vi "Dashboard Main.vi"() -> ()   [LabVIEW 2015]
uses:
  AnnieFramework/DoubleSolenoidAction.ctl
  AnnieFramework/CollectorAction.ctl
  AnnieFramework/CollectorWrapAction.ctl
  AnnieFramework/CatchAction.ctl
  AnnieFramework/AutoStates.ctl
  AnnieFramework/RollerAction.ctl
  AnnieFramework/AutoMode.ctl
  AnnieFramework/PassState.ctl
  AnnieFramework/HotGoalDetectType.ctl
  AnnieFramework/LowGoalState.ctl
  <vilib>/sound2/lvsound2.llb/Sound Data Format.ctl
  TabEnum.ctl
  <vilib>/event_ctls.llb/eventvkey.ctl
  <vilib>/Rock Robotics/WPI/Dashboard/WPI_DashboardLogging Global.vi
  KariFramework/CheckImageDistance.vi
  <vilib>/Utility/config.llb/Write Key (String).vi
  <vilib>/Utility/config.llb/Write Key (I32).vi
  <vilib>/Rock Robotics/Network Tables/NT Read Boolean.vi
  <vilib>/Utility/config.llb/NI_LVConfig.lvlib
  <vilib>/sound2/lvsound2.llb/Sound Input Read (DBL).vi
  <vilib>/Analysis/NI_AALPro.lvlib
  <vilib>/sound2/lvsound2.llb/Sampling Mode.ctl
panel:
  in  "Enable Vision":bool=TRUE
  out "Image Message":string="Timeout in Camera Communications"
  in  "Rec Mode":enum32{"Stop", "Record", "Playback"}(radio)
  in  "Dashboard Tab":T1(tab)
  in  "DisableKinect":bool=TRUE
  out "Version":string
  in  "XBox":bool
  in  "DisableLCD":bool=TRUE
  out "GroundPassState":T2
  in  "DisableRollerOut":bool=TRUE
  out "FrontSonar":dbl
  out "AtPressure":bool
  out "CatchState":T3
  out "CollectorWrapState":T4
  out "CollectorState":T5
  out "CollectorMotor":dbl
  out "ClapperState":T6
  out "RollerPneuState":T6
  out "FiringCylinder2":bool
  out "FiringCylinder1":bool
  out "Kicker":bool
  out "AutoDistanceDone?":bool
  out "BackSonar":dbl
  out "BottomLS":bool
  out "TopLS":bool
  in  "MaxMotorChange":dbl=1.5
  out "Error":bool
  out "Right Motor":dbl
  out "Left Motor":dbl
  in  "Camera Settings":T7={"Frame Rate"=30, "Compression"=30, "Size"=1} {"Frame Rate" scale=1.0..30.0; "Size" items=["640x480", "320x240", "160x120"]}
  out "Mode":T8(ring)=enum.""
  out "Camera IP":string="0.0.0.11"
  in  "DB Camera Config":bool
  out "fps":dbl format="%#.1g"
  out "Mbps":dbl format="%#.1g"
  out "Mbps 2":bool
  out "Pressure":i32
  out "RollerMotorState":T9
  in  "DisableServo":bool=TRUE
  out "ElevatedPassState":T2
  out "Arcade":bool
  out "TankDriveTime":dbl
  out "SonicShifter":bool
  out "StraightDrive":bool
  out "HalfDrive":bool
  out "ReverseDrive":bool
  out "LowGoalDumpState":T10
  out "KinectTriggered?":bool
  out "ServoAngle":dbl
  out "WebcamMatched? Copy":bool
  out "PitchDetected Copy":bool
  in  "PreScumbagWait":i32
  out "CheckGoalTime":u32
  in  "StartShootTime":i32=5000
  in  "DriveBackTime":i32=1000
  in  "DriveBackSpeed":dbl=-1.0
  in  "EndInLowGear?":bool=TRUE
  out "DriveElapsedTime":u32
  in  "AccelBackward":dbl=0.1
  in  "AccelForward":dbl=0.1
  in  "StartInLowGear?":bool=TRUE
  out "ShootTime":u32
  in  "BallSettleWait":i32=130
  in  "PreCheckGoalWait":i32=260
  in  "Slowdown":dbl=36.0
  in  "Brake":dbl=12.0
  in  "DriveDistance":dbl=36.0
  in  "DriveMinTime":i32=2000
  in  "DriveTimeout":i32=4000
  out "WasHot?":bool
  out "DriveTimeOut":bool
  out "CheckGoalTimedOut?":bool
  out "ElapsedTime":u32
  out "StateTime":u32
  out "CurrentState":T11
  out "RaiseArmTimedOut":bool
  out "LowerArmTimedOut":bool
  out "IDMatched?":bool
  in  "AutoID":i32=3061
  in  "AutoMode":T12=enum."OneBallCollector"
  in  "HotGoalType":T13
  in  "ResetSound?":bool
  out "Frequency":T14(graph)={"df"=0.0, "df"=2.205, "Power Spectrum (V^2 rms)"=array[5000 elements]}
  out "RawData":waveform(dbl)[](graph)=[{"t0"=timestamp(3478468008.2170343 s since 1904-01-01), "dt"=4.5351473922902495e-05, "Y"=array[10000 elements]}, {"t0"=timestamp(3478468008.2170343 s since 1904-01-01), "dt"=4.5351473922902495e-05, "Y"=array[10000 elements]}]
  out "MaxValue":dbl=1.242701184627817e-06 format="%#.5f"
  in  "Average":dbl=1.0
  in  "Freq Bandwidth":dbl=500.0 format="%#_13g"
  in  "Start Freq":dbl=4000.0 format="%#_13g"
  in  "SoundFormat":T15={"sample rate (S/s)"=22050.0, "number of channels"=2, "bits per sample"=16}
  in  "StopSoundDetect":bool
  in  "SoundCutoff":dbl=10.0 format="%#_13g"
  out "PitchDetected":bool
  in  "% Cutoff":dbl=0.5
  out "NumHot":i32
  out "NumProcessed":i32
  in  "NumSamples":i32=5
  out "ProcessImage?":bool
  in  "Finished?":bool
  in  "Hot?":bool
  in  "Score cutoff":dbl=0.5
  in  "Color System":u16(ring)=2 items=["RGB", "HSL", "HSV", "HSI"]
  out "Distance (ft)":dbl
  in  "Color Components":T16={"Hue"={112.0, 144.0}, "Sat"={202.0, 255.0}, "Val"={237.0, 255.0}} {"Val" scale=0.0..255.0; "Sat" scale=0.0..255.0; "Hue" scale=0.0..255.0 scale format="%#_3g"}
  out "LoopTime":u32=500
  in  "Calibrate?":bool
  in  "Reset?":bool
  in  "SaveCameraImage?":bool=TRUE
  in  "TestWebcam?":bool
  in  "RunWebcam?":bool
  out "WebcamImagesProcessed":i32
  in  "ResetWebcam?":bool
  in  "WebcamImages":i32=1
  in  "SaveWebcamImage?":bool
  out "WebcamMatched?":bool
  in  "WebcamStartTime (ms)":i32=2000
  in  "StopWebcam?":bool
  out "WebcamImage":T17(plugin-control)
  in  "height":i32=480
  in  "width":i32=640
  in  "driver":i32
  in  "Test Slider":dbl(slide) scale=0.0..100.0 scale format="%#_3g"
  in  "On/Off":bool caption="Solenoid"
  in  "Test Name":u16(ring) items=["Select the test to run...", "Example Test", "-------------------------------", "List of tests is built in robot code.", "Replace with your own automated tests."]
  in  "Test Tree":string(tree)
  in  "Motor":cluster{"Value":dbl, "Enable":bool} {"Value" scale=-1.0..1.0 scale format="%#_3g"}
  out "Progress":T18 {"Test Progress" scale=0.0..100.0}
  in  "Rev/Fwd":cluster{"Forward":bool, "Reverse":bool}
  in  "Test Ring":u16(ring) items=["Auto", "Fixed indoor", "Fixed outdoor 1", "Fixed outdoor 2", "Fixed fluorescent 1", "Fixed fluorescent 2", "Hold current"]
  in  "Listbox":i32(listbox)
  out "Tree":string(tree)
  out "ClosePressure":bool
  out "CloseDist":bool
  out "FarDist":bool
  out "Timer":u32
  in  "CountdownStartTime":u32=10
  in  "AutoLength":u32=10
  in  "TeleopLength":u32=140
  out "Status":T19(ring)
  in  "Beep?":bool=TRUE
  out "SoundFilePath":path
  out "Errors":T20(array[cluster])
  in  "Reset":bool
  out "Camera Image":T17(plugin-control)
  # "DRIVE"
  # "GENERAL"
  # "OUTPUT"
  # "CONFIG"
  # "DEPRECATED"
  # "COUNTDOWN"
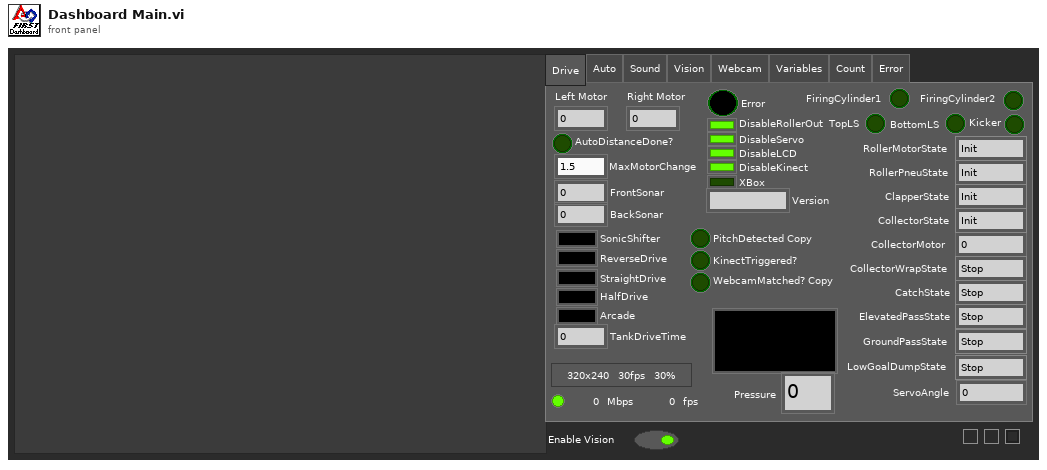
[diagram p1: front panel]
types:
  T1 = enum32{"Drive", "Auto", "Sound", "Vision", "Webcam", "Test", "Checklist", "Variables", "Count", "Error"}
  T2 = typedef "PassState.ctl" = enum16{"Stop", "Pass"}
  T3 = typedef "CatchAction.ctl" = enum16{"Stop", "PreCatch", "Catch"}
  T4 = typedef "CollectorWrapAction.ctl" = enum16{"Stop", "PreCollect", "Collect"}
  T5 = typedef "CollectorAction.ctl" = enum16{"Init", "Raise", "Lower", "Stop", "GetStatus"}
  T6 = typedef "DoubleSolenoidAction.ctl" = enum16{"Init", "Middle", "In", "Out"}
  T7 = cluster{"Frame Rate":i32, "Compression":i32, "Size":u16}
  T8 = enum8{"Tele-Op Disabled", "Tele-Op Enabled", "Auto Disabled", "Auto Enabled", "Test Disabled", "Test Enabled", ""}
  T9 = typedef "RollerAction.ctl" = enum16{"Init", "Off", "Forward", "Reverse"}
  T10 = typedef "LowGoalState.ctl" = enum16{"Stop", "Shoot"}
  T11 = typedef "AutoStates.ctl" = enum16{"Init", "LowerArmCheckGoal", "DriveBack", "Collect", "StopCollect", "LiftArm", "RaiseServo", "Drive", "ShootCollectorUp", "RaiseArm", "ShootCollectorDown", "Rotate1", "Rotate2", "Stop"}
  T12 = typedef "AutoMode.ctl" = enum16{"OneBallFront", "OneBallCollector", "TwoBallNormal", "TwoBallHot"}
  T13 = typedef "HotGoalDetectType.ctl" = enum16{"VisionTarget", "Kinect", "SoundDetect", "Webcam"}
  T14 = cluster{"df":dbl, "df":dbl, "Power Spectrum (V^2 rms)":dbl[]}
  T15 = typedef "Sound Data Format.ctl" = cluster{"sample rate (S/s)":dbl, "number of channels":i32, "bits per sample":i32}
  T16 = cluster{"Hue":cluster{dbl, dbl}, "Sat":cluster{dbl, dbl}, "Val":cluster{dbl, dbl}}
  T17 = typedef "IMAQ Image.ctl" = refnum<image>
  T18 = cluster{"Test Progress":u8, "Test Progress Text":string}
  T19 = enum8{"Disconnected", "E-Stop", "Disabled", "Enabled"}
  T20 = cluster{"status":bool, "code":i32, "location":string, "source":string}[]
  T21 = typedef "TabEnum.ctl" = enum32{"Drive", "Auto", "Sound", "Vision", "Webcam", "Variables", "Countdown", "Error"}
  T22 = typedef "Image Type" = u32
  T23 = typedef "Sampling Mode.ctl" = i32
  T24 = typedef "Sound Input Task ID.ctl" = u32
  T25 = typedef "NI_LVConfig.lvlib/Config Data RefNum.ctl" = refnum<k1>
  T26 = typedef "Sound Output Task ID.ctl" = u32
  T27 = cluster{"Digital Inputs":bool[], "Digital Outputs":bool[]}
  T28 = cluster{"Competition mode":bool, "Robot Link":bool, "Autonomous":bool, "Enabled":bool, "E-Stop":bool, "Simulated":bool, "TestMode":bool, "Docked Window":bool}
  T29 = typedef "CountdownAction.ctl" = enum16{"Start", "Reset", "Continue", "Idle"}
  T30 = cluster{"Boolean":bool, "Numeric":i32, "String":string, "String":string}[]
  T31 = cluster{cluster{dbl, dbl}, cluster{dbl, dbl}, cluster{dbl, dbl}}
  T32 = typedef "eventvkey.ctl" = enum16{"ASCII", "Enter", "Return", "Shift", "Ctrl", "Alt", "Cmd", "Opt", "Caps", "NumLock", "Clear", "Break", "Up", "Down", "Left", "Right", "Insert", "Delete", "Home", "End", "PageUp", "PageDown", "Escape", "Help", "Pause", "ScrollLock", "F1", "F2", "F3", "F4", "F5", "F6", "F7", "F8", "F9", "F10", "F11", "F12", "F13", "F14", "F15", "F16", "F17", "F18", "F19", "F20", "F21", "F22", "F23", "F24", "Play", "VolumeUp", "VolumeDown", "Mute", "Two Byte Char"}
  T33 = cluster{"Image Size":bool, "Image Type":bool, "Pixel Value":bool, "ROI Information":bool, "Zoom Factor":bool}
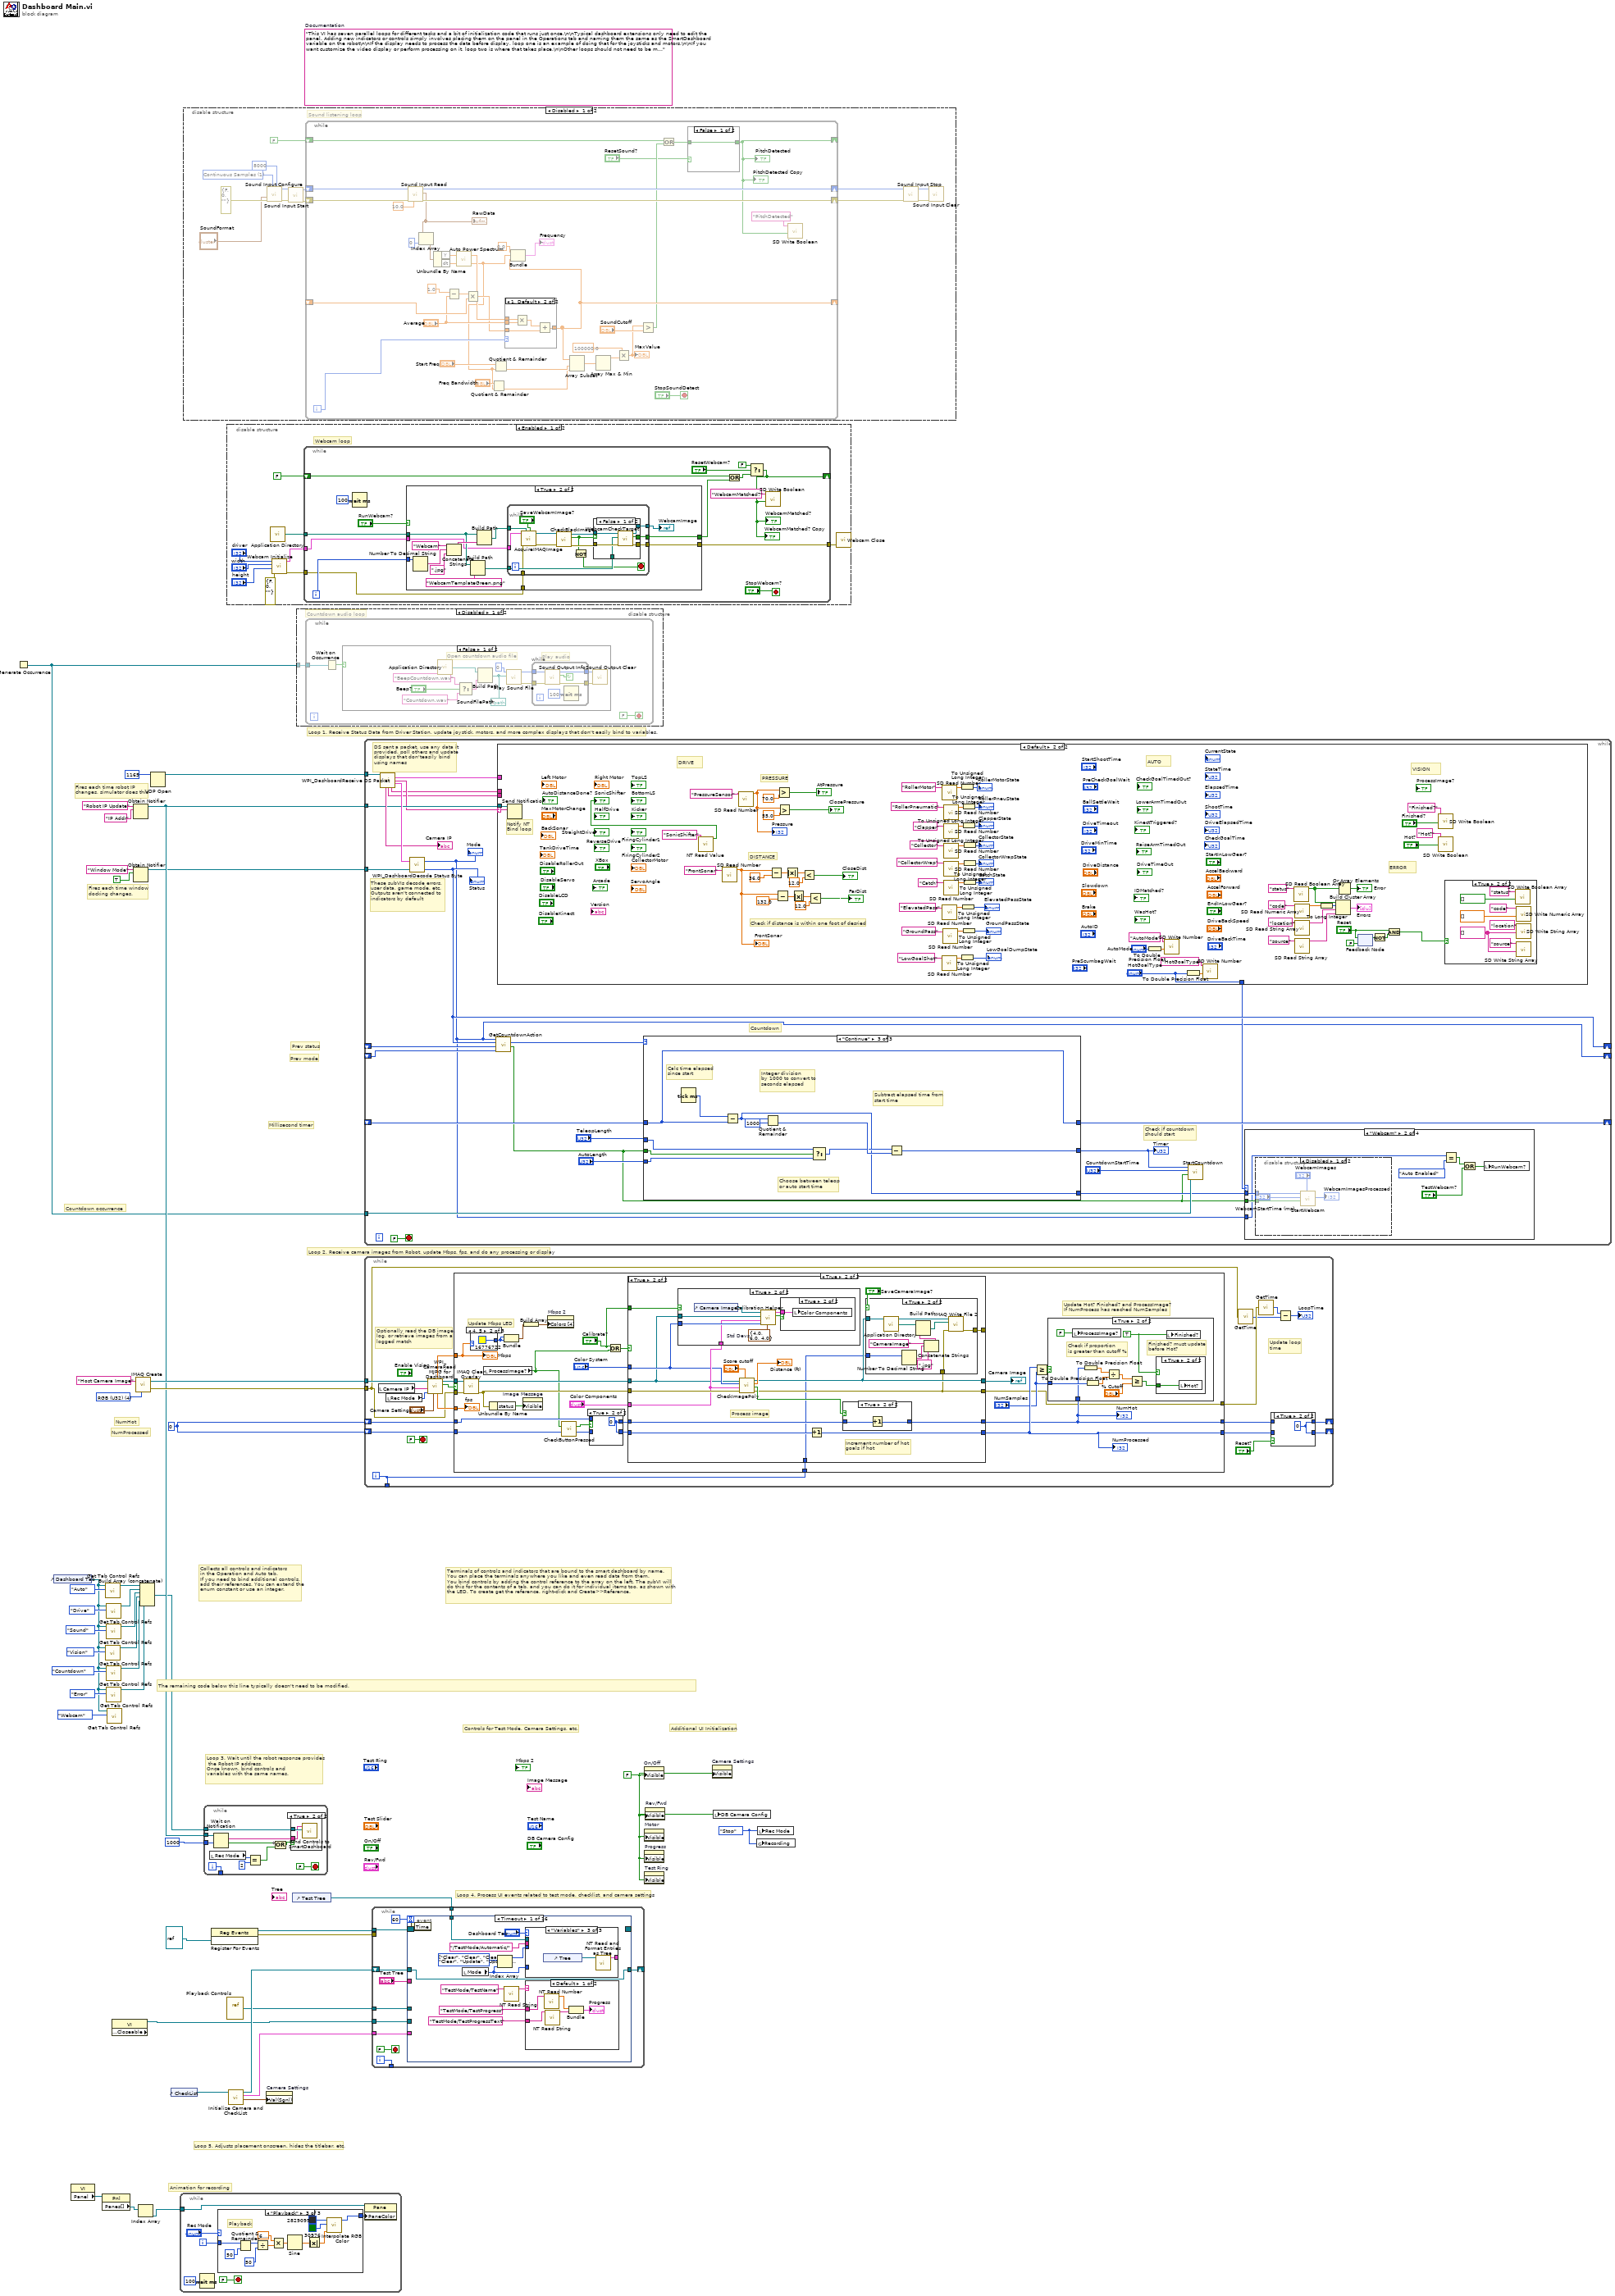
[diagram p0: block diagram]
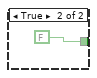
[diagram p4: hidden frame]
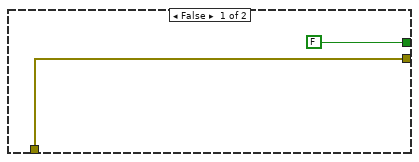
[diagram p7: hidden frame]
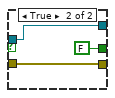
[diagram p8: hidden frame]
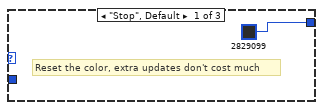
[diagram p10: hidden frame]
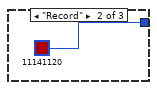
[diagram p11: hidden frame]
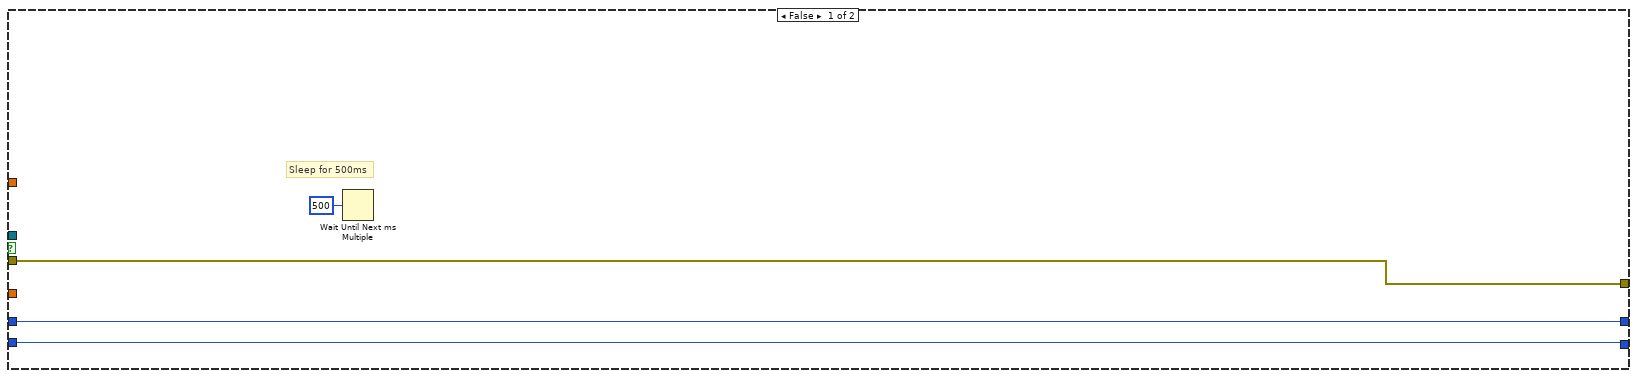
[diagram p14: hidden frame]
diagram:
  w13 = 0
  w19 = enum32{"Stop", "Record", "Playback"}."Stop" ("Rec Mode")
  w34 = FALSE ("Visible")
  (unwired) "This VI has seven parallel loops for different tasks and a bit of initialization code that runs just once.\n\nTypical dashboard extensions only need to edit the panel. Adding new indicators or controls simply involves placing them on the panel in the Operations tab and naming them the same as the SmartDashboard variable on the robot\n\nIf the display needs to process the data before display, loop one is an example of doing that for the joysticks and motors.\n\nIf you want customize the video display or perform processing on it, loop two is where that takes place.\n\nOther loops should not need to be modified. They are pretty standard, and document the task they perform."  # Documentation
  w43 = T22 4 items=["Grayscale (U8)", "Grayscale (I16)", "Grayscale (SGL)", "Complex (CSG)", "RGB (U32)", "HSL (U32)", "RGB (U64)"] ("Image Type")
  # "Prev mode"
  # "Countdown occurrence"
  # "Millisecond timer"
  # "Prev status"
  # "NumProcessed"
  # "NumHot"
  # "Controls for Test Mode, Camera Settings, etc."
  # "Additional UI Initialization"
  # "Animation for recording"
  # "Fires each time robot IP\nchanges, simulator does this"
  # "Fires each time window\ndocking changes."
  # "Collects all controls and indicators\nin the Operation and Auto tab.\nIf you need to bind additional controls,\nadd their references. You can extend the\nenum constant or use an integer."
  # "The remaining code below this line typically doesn't need to be modified."
  # "Loop 4. Process UI events related to test mode, checklist, and camera settings"
  # "Terminals of controls and indicators that are bound to the smart dashboard by name.\nYou can place the terminals anywhere you like and even read data from them.\nYou bind controls by adding the control reference to the array on the left. The subVI will\ndo this for the contents of a tab, and you can do it for individual items too, as shown with\nthe LED. To create get the reference, right-click and Create>>Reference."
  # "Loop 3. Wait until the robot response provides\n the Robot IP address.\nOnce known, bind controls and\nvariables with the same names."
  # "Loop 5. Adjusts placement onscreen, hides the titlebar, etc."
  # "Loop 1. Receive Status Data from Driver Station, update joystick, motors, and more complex displays that don't easily bind to variables."
  # "Loop 2. Receive camera images from Robot, update Mbps, fps, and do any processing or display"
  n1 = Generate Occurrence() -> (w12:refnum<k4>)
  n2 = control-ref of="Dashboard Tab"() -> (w2:refnum<vi>)
  n3 = property class="VI"() -> ("Panel"=w28:refnum<vi>)  [unwired: 2 in, 2 out]
  n4 = property class="Pnl"(reference=w28) -> ("Panes[]"=w29:refnum<vi>[])  [unwired: 1 in, 2 out]
  n5 = call <vilib>:"Get Tab Control Refs.vi"("Page Index"=TabEnum."Auto" ("Dashboard Tab"), "TabControl in"=w2) -> ("ControlsOnPage"=w17:refnum<vi>[])  [unwired: 9 in]
  n6 = call <vilib>:"Get Tab Control Refs.vi"("Page Index"=TabEnum."Vision" ("Dashboard Tab"), "TabControl in"=w2) -> ("ControlsOnPage"=w5:refnum<vi>[])  [unwired: 9 in]
  n7 = call <vilib>:"Get Tab Control Refs.vi"("Page Index"=TabEnum."Drive" ("Dashboard Tab"), "TabControl in"=w2) -> ("ControlsOnPage"=w14:refnum<vi>[])  [unwired: 9 in]
  n8 = call <vilib>:"Get Tab Control Refs.vi"("Page Index"=TabEnum."Sound" ("Dashboard Tab"), "TabControl in"=w2) -> ("ControlsOnPage"=w6:refnum<vi>[])  [unwired: 9 in]
  n9 = call <vilib>:"Get Tab Control Refs.vi"("Page Index"=TabEnum."Countdown" ("Dashboard Tab"), "TabControl in"=w2) -> ("ControlsOnPage"=w4:refnum<vi>[])  [unwired: 9 in]
  n10 = call <vilib>:"Get Tab Control Refs.vi"("Page Index"=TabEnum."Error" ("Dashboard Tab"), "TabControl in"=w2) -> ("ControlsOnPage"=w3:refnum<vi>[])  [unwired: 9 in]
  n11 = call <vilib>:"Get Tab Control Refs.vi"("Page Index"=TabEnum."Webcam" ("Dashboard Tab"), "TabControl in"=w2) -> ()  [unwired: 9 in, 1 out]
  n12 = property class="VI" props=["Front Panel.Closeable"]() -> (reference out=w18:refnum<vi>)  [unwired: 2 in, 2 out]
  n13 = Obtain Notifier(name (unnamed)="Robot IP Update", notification data type="IP Addr" ("name (unnamed)")) -> (notifier out=w37:refnum<notifier>)  [unwired: 2 in, 2 out]
  n14 = Obtain Notifier(name (unnamed)="Window Mode", notification data type=TRUE) -> (notifier out=w21:refnum<notifier>)  [unwired: 2 in, 2 out]
  n15 = call "IMAQ Create"("Image Name"="Host Camera Image", "Image Type"=w43) -> ("New Image"=w41:T17, "error out"=w40:errorcluster)  [unwired: 2 in, 1 out]
  n16 = Index Array(array=w29) -> (element=w27:refnum<vi>)  [unwired: 1 in]
  n17 = Build Array (concatenate)(w17, w14, w6, w5, w4, w3) -> (w16:refnum<vi>[])
  n18 = UDP Open(11:u16 1165 ("port")) -> (port=w44:refnum<k16>)  [unwired: 2 in, 4 out]
  n19 = control-ref of="CheckList"() -> (w20:refnum<vi>)
  n20 = while {
    tunnel: w27 -> [w47]
    i -> [w50]
    stop <- FALSE stop-if-true
    n21 = Wait (ms)(milliseconds to wait=u32 100) -> ()  [unwired: 1 out]
    n22 = case shown="\"Playback\"" "Rec Mode" {
      tunnel: w50 -> [_ _ w65]
      tunnel: [u32 2829099 ("Base Color") u32 11141120 ("Target Color") w54] -> w46
      frame "Stop", Default {
        # "Reset the color, extra updates don't cost much"
      }
      frame "Record" {
      }
      frame "Playback" {
        # "Playback"
        n23 = Quotient & Remainder(x=w65, y=u32 50 ("milliseconds to wait")) -> (x-y*floor(x/y)=w61:u32)  [unwired: 1 out]
        n24 = Divide(x=w61, y=u32 50 ("milliseconds to wait")) -> (x/y=w58:dbl)
        n25 = Multiply(x=6.283185307179586, y=w58) -> (x*y=w63:dbl)
        n26 = Sine(x=w63) -> (sin(x)=w62:dbl)
        n27 = Absolute Value(x=w62) -> (abs(x)=w55:dbl)
        n28 = call "Interpolate RGB Color.vi"("Proportion"=w55, "Target Color"=u32 30976, "Base Color"=u32 2829099) -> ("Result Color"=w54:u32)  [unwired: 8 in]
      }
    }
    n29 = property class="Pane"(reference=w47, "PaneColor"=w46) -> ()  [unwired: 1 in, 2 out]
  }
  n30 = disable-structure shown="Disabled" {
    frame Disabled {
      w77 = T23 1 items=["Finite Samples", "Continuous Samples"] ("sample mode")
      # "Sound listening loop"
      n31 = call <vilib>:"Sound Input Configure.vi"("number of samples/ch"=8000, "sample mode"=w77, "error in (no error)"=errorcluster {"status"=FALSE, "code"=0, "source"=""}, "sound format"="SoundFormat") -> ("error out"=w74:errorcluster, "task ID"=w75:T24)  [unwired: 6 in]
      n32 = call <vilib>:"Sound Input Start.vi"("error in (no error)"=w74, "task ID"=w75) -> ("error out"=w73:errorcluster, "task ID out"=w72:T24)  [unwired: 8 in]
      n33 = while {
        shift-right: [w111] -> w71
        shift-left: w73 -> [w113]
        shift-right: [w112] -> w70
        shift-left: w72 -> [w114]
        shift-right: [w108] -> _
        shift-left: _ -> [w110]
        shift-right: [w79] -> _
        shift-left: FALSE -> [w84]
        i -> [w109]
        stop <- "StopSoundDetect" stop-if-true
        n34 = call-poly <vilib>:"Sound Input Read.vi"("timeout (sec)"=10.0, "error in (no error)"=w113, "task ID"=w114) -> ("error out"=w111:errorcluster, "data"=w106:waveform(dbl)[], "task ID out"=w112:T24)  [unwired: 6 in]
        "RawData" <- w106
        n35 = Index Array(array=w106, index=0) -> (element=w102:waveform(dbl))
        n36 = Unbundle By Name(w102) -> ("Y"=w103:dbl[], "dt"=w100:dbl)
        n37 = Subtract(x=1.0, y="Average") -> (x-y=w96:dbl)
        n38 = call <vilib>:"Auto Power Spectrum.vi"("dt"=w100, "Signal (V)"=w103) -> ("df"=w92:dbl, "Power Spectrum (V^2 rms)"=w99:dbl[])
        n39 = Multiply(x=w96, y=w110) -> (x*y=w95:dbl[])
        n40 = Quotient & Remainder(x="Freq Bandwidth", y=w92) -> (floor(x/y)=w90:dbl)  [unwired: 1 out]
        n41 = Quotient & Remainder(x="Start Freq", y=w92) -> (floor(x/y)=w91:dbl)  [unwired: 1 out]
        n42 = case shown="1, Default" w109 {
          tunnel: w99 -> [w118 w123]
          tunnel: "Average" -> [_ w122]
          tunnel: w95 -> [_ w120]
          tunnel: [w118 w119] -> w108
          frame 0 {
          }
          frame 1, Default {
            n43 = Multiply(x=w123, y=w122) -> (x*y=w121:dbl[])
            n44 = Add(x=w121, y=w120) -> (x+y=w119:dbl[])
          }
        }
        n45 = Bundle("df"=0.0, "df"=w92, "Power Spectrum (V^2 rms)"=w108) -> (→"Frequency":T14)  [unwired: 1 in]
        n46 = Array Subset(array=w108, index=w91, length=w90) -> (w89:dbl[])
        n47 = Array Max & Min(array=w89) -> (max value=w88:dbl)  [unwired: 3 out]
        n48 = Multiply(x=100000.0, y=w88) -> (x*y=w85:dbl)
        "MaxValue" <- w85
        n49 = Greater?(x=w85, y="SoundCutoff") -> (0:w83:bool)
        n50 = Or(x=w84, y=w83) -> (x .or. y?=w82:bool)
        n51 = case shown="False" "ResetSound?" {
          tunnel: w82 -> [w116 _]
          tunnel: [w116 FALSE] -> w79
          frame False {
          }
          frame True {
          }
        }
        "PitchDetected" <- w79
        "PitchDetected Copy" <- w79
        n52 = call <vilib>:"SD Write Boolean.vi"("Boolean"=w79, "Name"="PitchDetected") -> ()  [unwired: 8 in, 2 out]
      }
      n53 = call <vilib>:"Sound Input Stop.vi"("error in (no error)"=w71, "task ID"=w70) -> ("error out"=w69:errorcluster, "task ID out"=w68:T24)  [unwired: 8 in]
      n54 = call <vilib>:"Sound Input Clear.vi"("error in (no error)"=w69, "task ID"=w68) -> ()  [unwired: 9 in, 1 out]
    }
    frame Enabled {
    }
  }
  n55 = while {
    tunnel: w16 -> [w134]
    tunnel: w37 -> [w132]
    tunnel: [w130] -> _
    tunnel: u32 1000 ("milliseconds to wait") -> [w129]
    i -> [w130]
    stop <- FALSE stop-if-true
    n56 = local read "Rec Mode"() -> (w125:enum32{"Stop", "Record", "Playback"})
    n57 = Wait on Notification(notifier=w132, timeout in ms (-1)=w129) -> (notification=w131:string, timed out?=w127:bool)  [unwired: 2 in, 2 out]
    n58 = Equal?(x=w125, y=u16 2 ("Rec Mode")) -> (x = y?=w126:bool)
    n59 = Compound Arithmetic op=OR(invert w127, w126) -> (w128:bool)
    n60 = case shown="True" w128 {
      tunnel: w134 -> [_ w136]
      tunnel: w131 -> [_ w135]
      frame False {
      }
      frame True {
        n61 = call <vilib>:"Bind Controls to SmartDashboard.vi"("Bound Control Refs"=w136, "Server IP Address"=w135) -> ()  [unwired: 10 in]
      }
    }
  }
  n62 = register-events(refnum<vi> refnum) -> (reference out=w25:refnum<event-registration>, error out=w24:errorcluster)  [unwired: 2 in]
  n63 = disable-structure shown="Enabled" {
    frame Enabled {
      # "Webcam loop"
      n64 = call <vilib>:"Application Directory.vi"() -> ("Application Directory"=w137:path)
      n65 = call "Webcam Initialize.vi"("error in"=errorcluster {"status"=FALSE, "code"=0, "source"=""}, "height (240)"="height", "width (320)"="width", "driver (0)"="driver") -> ("error out"=w140:errorcluster, "webcam image out"=w141:cluster{"image":u8[], "width":i32, "height":i32})  [unwired: 4 in, 1 out]
      n66 = while {
        tunnel: w137 -> [w160]
        tunnel: w141 -> [w158]
        tunnel: w140 -> [w157]
        tunnel: [w156] -> w139
        shift-right: [w146] -> _
        shift-left: FALSE -> [w152]
        i -> [w159]
        stop <- "StopWebcam?" stop-if-true
        n67 = Wait (ms)(milliseconds to wait=u32 100) -> ()  [unwired: 1 out]
        n68 = case shown="True" "RunWebcam?" {
          tunnel: [w161 w176] -> w156
          tunnel: [FALSE ("MatchFound?") w175] -> w151
          tunnel: w159 -> [_ w173]
          tunnel: w160 -> [_ w168]
          tunnel: w158 -> [_ w165]
          tunnel: w157 -> [w161 w164]
          frame False {
          }
          frame True {
            n69 = Number To Decimal String(number=w173) -> (decimal integer string=w172:string)  [unwired: 1 in]
            n70 = Concatenate Strings("Webcam", w172, ".jpg" ("string")) -> (w171:string)
            n71 = Build Path(base path=w168, name or relative path="WebcamTemplateGreen.png") -> (appended path=w167:path)
            n72 = Build Path(base path=w168, name or relative path=w171) -> (appended path=w170:path)
            n73 = while {
              tunnel: [w190] -> w176
              tunnel: [w189] -> w175
              tunnel: w170 -> [w188]
              tunnel: w167 -> [w186]
              tunnel: w165 -> [w179]
              tunnel: w164 -> [w178]
              tunnel: [w177] -> w163
              stop <- w180 stop-if-true
              n74 = call "AcquireIMAQImage.vi"("ImagePath"=w188, "SaveToDisk?"="SaveWebcamImage?", "error in"=w178, "webcam image in"=w179) -> ("error out"=w185:errorcluster, "ImageOut"=w183:T17)  [unwired: 6 in]
              n75 = call "CheckBlackImage.vi"("error in"=w185, "Image In"=w183) -> ("error out"=w184:errorcluster, "Black?"=w181:bool, "Image Out"=w182:T17)  [unwired: 7 in]
              n76 = Not(x=w181) -> (.not. x?=w180:bool)
              n77 = case shown="False" w181 {
                tunnel: w182 -> [w196 w197]
                tunnel: w184 -> [w195 w199]
                tunnel: [w194 w199] -> w190
                tunnel: [w193 FALSE ("MatchFound?")] -> w189
                tunnel: w186 -> [w192 _]
                tunnel: [w191 w197] -> w177
                frame False {
                  n78 = call "WebcamCheckTarget.vi"("error in"=w195, "TemplatePath"=w192, "ImageIn"=w196) -> ("error out"=w194:errorcluster, "MatchFound?"=w193:bool, "Image Out"=w191:T17)  [unwired: 6 in]
                }
                frame True {
                }
              }
            }
            "WebcamImage" <- w163
          }
        }
        n79 = Or(x=w152, y=w151) -> (x .or. y?=w149:bool)
        n80 = Select(t=FALSE, s="ResetWebcam?", f=w149) -> (s? t:f=w146:bool)
        "WebcamMatched?" <- w146
        "WebcamMatched? Copy" <- w146
        n81 = call <vilib>:"SD Write Boolean.vi"("Boolean"=w146, "Name"="WebcamMatched?") -> ()  [unwired: 8 in, 2 out]
      }
      n82 = call "Webcam Close.vi"("error in"=w139) -> ()  [unwired: 9 in, 1 out]
    }
    frame Disabled {
    }
  }
  n83 = vi-ref "Playback Controls.vi"() -> (w26:refnum<vi>)
  n84 = call "Initialize Camera and CheckList.vi"("ListBox in"=w20) -> ("Cluster"=w32:cluster{"value":i32, "value":i32, "index":i32}, "Array"=w33:cluster{string[]}[], "File Refnum"=w31:T25)  [unwired: 8 in]
  n85 = property on="Camera Settings" class="Clust (strict)"("Val(Sgnl)"=w32) -> ()  [unwired: 2 in, 2 out]
  n86 = control-ref of="Test Tree"() -> (w30:refnum<vi>)
  n87 = disable-structure shown="Disabled" {
    disable-tunnel: w12 -> [w200 _]
    frame Disabled {
      # "Countdown audio loop"
      n88 = while {
        tunnel: w200 -> [w201]
        stop <- FALSE stop-if-true
        n89 = Wait on Occurrence(2:w201) -> (0:w203:bool)  [unwired: 2 in]
        n90 = case shown="False" w203 {
          frame False {
            # "Play audio"
            # "Open countdown audio file"
            n91 = call <vilib>:"Application Directory.vi"() -> ("Application Directory"=w204:path)
            n92 = Select(t="BeepCountdown.wav" ("name or relative path"), s="Beep?", f="Countdown.wav" ("name or relative path")) -> (s? t:f=w206:string)
            n93 = Build Path(base path=w204, name or relative path=w206) -> (appended path=w205:path)
            "SoundFilePath" <- w205
            n94 = call <vilib>:"Play Sound File.vi"("path"=w205, "device ID"=u32 0) -> ("error out"=w213:errorcluster, "task ID"=w212:T26)  [unwired: 8 in]
            n95 = while {
              tunnel: w213 -> [w215]
              tunnel: w212 -> [w219]
              tunnel: [w218] -> w211
              tunnel: [w216] -> w210
              stop <- w217 continue-if-true
              n96 = call <vilib>:"Sound Output Info.vi"("error in (no error)"=w215, "task ID"=w219) -> ("error out"=w216:errorcluster, "is playing?"=w217:bool, "task ID out"=w218:T26)  [unwired: 6 in, 1 out]
              n97 = Wait (ms)(milliseconds to wait=u32 100) -> ()  [unwired: 1 out]
            }
            n98 = call <vilib>:"Sound Output Clear.vi"("error in (no error)"=w210, "task ID"=w211) -> ()  [unwired: 9 in, 1 out]
          }
          frame True {
          }
        }
      }
    }
    frame Enabled {
    }
  }
  n99 = while {
    tunnel: w44 -> [w243]
    tunnel: w37 -> [w240]
    tunnel: w21 -> [w242]
    shift-right: [w235] -> _
    shift-left: _ -> [w234]
    shift-right: [w232] -> _
    shift-left: _ -> [w231]
    tunnel: w12 -> [w226]
    shift-right: [w221] -> _
    shift-left: _ -> [w223]
    stop <- FALSE stop-if-true
    # "Check if countdown\nshould start"
    # "Countdown"
    # "DS sent a packet. use any data it\nprovided, poll others and update\ndisplays that don'teasily bind\nusing names"
    # "These subVIs decode errors, user data, game mode, etc.\nOutputs aren't connected to indicators by default"
    n100 = call <vilib>:"WPI_DashboardReceive DS Packet.vi"("Recv Socket"=w243) -> ("Driver Station"=w236:T27, "Robot IP Address"=w239:string, "Status"=w244:T28, "Camera IP Address"=→"Camera IP":string, "Low Priority User Data"=w238:string, "High Priority User Data"=w237:string)  [unwired: 2 in, 7 out]
    n101 = call <vilib>:"WPI_DashboardDecode Status Byte.vi"("Window Mode Notifier"=w242, "Status"=w244) -> ("Status"=w235:T19, "Mode"=w221:T8)
    "Mode" <- w221
    "Status" <- w235
    n102 = call "GetCountdownAction.vi"("PrevMode"=w223, "PrevStatus"=w234, "CurrentStatus"=w235, "CurrentMode"=w221) -> ("Teleop?"=w224:bool, "Action"=w233:T29)  [unwired: 6 in]
    n103 = case shown="Default" w239 {
      selector: w239 -> [_ w350]
      tunnel: w240 -> [_ w351]
      tunnel: w238 -> [_ _]
      tunnel: w237 -> [_ _]
      tunnel: w236 -> [_ _]
      tunnel: [_ "HotGoalType"] -> w222
      frame "0.0.0.0" {
        # "DS not sending packets, or no robot exists yet.\nDon't poll the variables"
      }
      frame Default {
        # "Check if distance is within one foot of desried"
        # "ERROR"
        # "DISTANCE"
        # "PRESSURE"
        # "VISION"
        # "AUTO"
        # "DRIVE"
        # "Notify NT\nBind loop"
        n104 = Send Notification(notification=w350, notifier=w351) -> ()  [unwired: 1 in, 2 out]
        n105 = call-poly <vilib>:"NT Read Value.vi"("Name"="SonicShifter") -> ("Boolean"=→"SonicShifter":bool)  [unwired: 9 in, 1 out]
        n106 = call <vilib>:"SD Read Number.vi"("Name"="FrontSonar") -> ("Numeric"=w301:dbl)  [unwired: 8 in, 2 out]
        "FrontSonar" <- w301
        n107 = call <vilib>:"SD Read Number.vi"("Name"="PressureSensor") -> ("Numeric"=w300:dbl)  [unwired: 8 in, 2 out]
        "Pressure" <- w300
        n108 = Subtract(x=w301, y=36.0) -> (x-y=w308:dbl)
        n109 = Subtract(x=w301, y=132.0) -> (x-y=w303:dbl)
        n110 = Greater?(x=w300, y=70.0) -> (0:→"AtPressure":bool)
        n111 = Greater?(x=w300, y=55.0) -> (0:→"ClosePressure":bool)
        n112 = Absolute Value(x=w308) -> (abs(x)=w307:dbl)
        n113 = Absolute Value(x=w303) -> (abs(x)=w304:dbl)
        n114 = Less?(x=w307, y=12.0) -> (x < y?=→"CloseDist":bool)
        n115 = Less?(x=w304, y=12.0) -> (x < y?=→"FarDist":bool)
        n116 = call <vilib>:"SD Read Number.vi"("Name"="LowGoalShot") -> ("Numeric"=w284:dbl)  [unwired: 8 in, 2 out]
        n117 = call <vilib>:"SD Read Number.vi"("Name"="RollerMotor") -> ("Numeric"=w298:dbl)  [unwired: 8 in, 2 out]
        n118 = call <vilib>:"SD Read Number.vi"("Name"="ElevatedPass") -> ("Numeric"=w292:dbl)  [unwired: 8 in, 2 out]
        n119 = call <vilib>:"SD Read Number.vi"("Name"="GroundPass") -> ("Numeric"=w291:dbl)  [unwired: 8 in, 2 out]
        n120 = call <vilib>:"SD Read Number.vi"("Name"="RollerPneumatic") -> ("Numeric"=w328:dbl)  [unwired: 8 in, 2 out]
        n121 = call <vilib>:"SD Read Number.vi"("Name"="Clapper") -> ("Numeric"=w326:dbl)  [unwired: 8 in, 2 out]
        n122 = call <vilib>:"SD Read Number.vi"("Name"="Collector") -> ("Numeric"=w323:dbl)  [unwired: 8 in, 2 out]
        n123 = call <vilib>:"SD Read Number.vi"("Name"="CollectorWrap") -> ("Numeric"=w320:dbl)  [unwired: 8 in, 2 out]
        n124 = call <vilib>:"SD Read Number.vi"("Name"="Catch") -> ("Numeric"=w317:dbl)  [unwired: 8 in, 2 out]
        n125 = To Unsigned Long Integer(number=w298) -> (unsigned 32bit integer=→"RollerMotorState":u32)
        n126 = To Unsigned Long Integer(number=w284) -> (unsigned 32bit integer=→"LowGoalDumpState":u32)
        n127 = To Unsigned Long Integer(number=w292) -> (unsigned 32bit integer=→"ElevatedPassState":u32)
        n128 = To Unsigned Long Integer(number=w328) -> (unsigned 32bit integer=→"RollerPneuState":u32)
        n129 = To Unsigned Long Integer(number=w326) -> (unsigned 32bit integer=→"ClapperState":u32)
        n130 = To Unsigned Long Integer(number=w291) -> (unsigned 32bit integer=→"GroundPassState":u32)
        n131 = To Unsigned Long Integer(number=w323) -> (unsigned 32bit integer=→"CollectorState":u32)
        n132 = To Unsigned Long Integer(number=w320) -> (unsigned 32bit integer=→"CollectorWrapState":u32)
        n133 = To Unsigned Long Integer(number=w317) -> (unsigned 32bit integer=→"CatchState":u32)
        n134 = To Double Precision Float(number="AutoMode") -> (double precision float=w294:dbl)
        n135 = call <vilib>:"SD Write Number.vi"("Numeric"=w294, "Name"="AutoMode") -> ()  [unwired: 8 in, 2 out]
        n136 = To Double Precision Float(number="HotGoalType") -> (double precision float=w287:dbl)
        n137 = call <vilib>:"SD Write Number.vi"("Numeric"=w287, "Name"="HotGoalType") -> ()  [unwired: 8 in, 2 out]
        n138 = call <vilib>:"SD Read Boolean Array.vi"("Name"="status") -> ("Boolean Array"=w339:bool[])  [unwired: 8 in, 2 out]
        n139 = call <vilib>:"SD Read Numeric Array.vi"("Name"="code") -> ("Numeric Array"=w338:dbl[])  [unwired: 8 in, 2 out]
        n140 = call <vilib>:"SD Read String Array.vi"("Name"="location") -> ("String Array"=w337:string[])  [unwired: 9 in, 1 out]
        n141 = call <vilib>:"SD Read String Array.vi"("Name"="source") -> ("String Array"=w336:string[])  [unwired: 9 in, 1 out]
        n142 = To Long Integer(number=w338) -> (32bit integer=w344:i32[])
        n143 = Build Cluster Array(w339, w344, w337, w336) -> (→"Errors":T30)
        n144 = Or Array Elements(Boolean array=w339) -> (logical OR=→"Error":bool)
        n145 = feedback #1(FALSE ("Reset")) -> (w347:bool)
        n146 = feedback-in #1("Reset") -> ()
        n147 = Not(x=w347) -> (.not. x?=w346:bool)
        n148 = And(x="Reset", y=w346) -> (x .and. y?=w345:bool)
        n149 = call <vilib>:"SD Write Boolean.vi"("Boolean"="Finished?", "Name"="Finished?") -> ()  [unwired: 8 in, 2 out]
        n150 = call <vilib>:"SD Write Boolean.vi"("Boolean"="Hot?", "Name"="Hot?") -> ()  [unwired: 8 in, 2 out]
        n151 = case shown="True" w345 {
          frame False {
          }
          frame True {
            w352 = string[] [] ("String Array")
            n152 = call <vilib>:"SD Write Boolean Array.vi"("Boolean Array"=bool[] [], "Name"="status") -> ()  [unwired: 8 in, 2 out]
            n153 = call <vilib>:"SD Write Numeric Array.vi"("Numeric Array"=dbl[] [], "Name"="code") -> ()  [unwired: 8 in, 2 out]
            n154 = call <vilib>:"SD Write String Array.vi"("String Array"=w352, "Name"="location") -> ()  [unwired: 8 in, 2 out]
            n155 = call <vilib>:"SD Write String Array.vi"("String Array"=w352, "Name"="source") -> ()  [unwired: 8 in, 2 out]
          }
        }
      }
    }
    n156 = case shown="\"Continue\"" w233 {
      tunnel: "TeleopLength" -> [w261 _ w274]
      tunnel: "AutoLength" -> [w260 _ w273]
      tunnel: [w264 w265 w272] -> w228
      tunnel: [w263 w266 w271] -> w232
      tunnel: w231 -> [_ w266 w271]
      tunnel: w224 -> [w262 _ w275]
      tunnel: [u32 0 ("millisecond timer value") w265 w267] -> w225
      frame "Start", Default {
        # "Choose between auto and teleop start times"
        n157 = Select(t=w261, s=w262, f=w260) -> (s? t:f=w264:u32)
        n158 = Tick Count (ms)() -> (millisecond timer value=w263:u32)
      }
      frame "Reset", "Idle" {
        w265 = u32 0 ("AutoStartTime")
      }
      frame "Continue" {
        # "Subtract elapsed time from\nstart time"
        # "Choose between teleop\nor auto start time"
        # "Integer division\nby 1000 to convert to\nseconds elapsed"
        # "Calc time elapsed\nsince start"
        n159 = Tick Count (ms)() -> (millisecond timer value=w268:u32)
        n160 = Subtract(x=w268, y=w271) -> (x-y=w267:u32)
        n161 = Quotient & Remainder(x=w267, y=u32 1000) -> (floor(x/y)=w270:u32)  [unwired: 1 out]
        n162 = Select(t=w274, s=w275, f=w273) -> (s? t:f=w269:u32)
        n163 = Subtract(x=w269, y=w270) -> (x-y=w272:u32)
      }
    }
    "Timer" <- w228
    n164 = call "StartCountdown.vi"("CountdownOccurrence"=w226, "Teleop?"=w224, "CountdownStartTime"="CountdownStartTime", "Time"=w228) -> ()  [unwired: 8 in]
    n165 = case shown="\"Webcam\"" w222 {
      tunnel: w225 -> [_ w252 _ _]
      tunnel: w224 -> [_ w251 _ _]
      tunnel: w221 -> [_ w250 _ _]
      frame "VisionTarget", Default {
      }
      frame "Webcam" {
        n166 = disable-structure shown="Disabled" {
          disable-tunnel: w252 -> [w258 _]
          disable-tunnel: w251 -> [w257 _]
          frame Disabled {
            n167 = call "StartWebcam.vi"("NumWebcamImages"="WebcamImages", "Teleop?"=w257, "WebcamStartTime (ms)"="WebcamStartTime (ms)", "ElapsedTime (ms)"=w258) -> ("WebcamImagesProcessed"=→"WebcamImagesProcessed":i32, "ResetWebcam?"=w254:bool)  [unwired: 6 in]
          }
          frame Enabled {
          }
        }
        n168 = Equal?(x=w250, y=T8."Auto Enabled") -> (x = y?=w248:bool)
        n169 = Or(x=w248, y="TestWebcam?") -> (x .or. y?=w246:bool)
        n170 = local write "RunWebcam?"(w246) -> ()
      }
      frame "Kinect" {
      }
      frame "SoundDetect" {
      }
    }
  }
  n171 = while {
    tunnel: w41 -> [w379]
    tunnel: w40 -> [w365]
    tunnel: [w359] -> _
    shift-right: [w360] -> _
    shift-left: w13 -> [w370]
    shift-right: [w361] -> _
    shift-left: w13 -> [w371]
    i -> [w359]
    stop <- FALSE stop-if-true
    # "Update loop\ntime"
    # "Optionally read the DB image,\nlog, or retrieve images from a\nlogged match"
    n172 = local read "Camera IP"() -> (w373:string)
    n173 = local read "Rec Mode"() -> (w372:enum32{"Stop", "Record", "Playback"})
    n174 = call <vilib>:"WPI_CameraRead MJPG for Dashboard.vi"("Camera Settings"="Camera Settings", "Rec Mode"=w372, "Camera IP"=w373, "Refnum in"=w379) -> ("Active"=w377:bool, "Refnum out"=w378:T17, "FPS"=w376:dbl, "Bandwidth (Mbps)"=w375:dbl)  [unwired: 4 in]
    n175 = case shown="True" w377 {
      tunnel: w378 -> [_ w410]
      tunnel: w375 -> [_ w409]
      tunnel: w376 -> [_ w408]
      tunnel: w371 -> [w385 w398]
      tunnel: w370 -> [w386 w397]
      tunnel: [w386 w403] -> w363
      tunnel: [w385 w402] -> w362
      tunnel: [w384 w400] -> w368
      tunnel: w365 -> [w384 w399]
      tunnel: w359 -> [_ w388]
      frame False {
        # "Sleep for 500ms"
        n176 = Wait Until Next ms Multiple(millisecond multiple=u32 500) -> ()  [unwired: 1 out]
      }
      frame True {
        # "Update Hot? Finished? and ProcessImage?\nIf NumProcess has reached NumSamples"
        # "Update Mbps LED"
        n177 = call "IMAQ Clear Overlay"("error in (no error)"=w399, "Image"=w410) -> ("error out"=w405:errorcluster, "Image Out"=w407:T17)  [unwired: 1 in, 7 out]
        n178 = case shown="4, 5" w409 {
          tunnel: [u32 6618880 ("Color Box") u32 16776722 ("Color Box") u32 16716800 ("Color Box")] -> w411
          frame Default {
          }
          frame 4, 5 {
          }
          frame 6.. {
          }
        }
        n179 = local read "ProcessImage?"() -> (w390:bool)
        n180 = Unbundle By Name(w405) -> ("status"=w414:bool)
        n181 = Bundle("Color Box"=w411, "Color Box"=w411) -> (w413:cluster{"Color Box":u32, "Color Box":u32})  [unwired: 1 out]
        n182 = property on="Image Message" class="Str"("Visible"=w414) -> ()  [unwired: 2 in, 2 out]
        n183 = Build Array(w413) -> (w412:cluster{"Color Box":u32, "Color Box":u32}[])
        n184 = property on="Mbps 2" class="Bool (strict)"("Colors [4]"=w412) -> ()  [unwired: 2 in, 2 out]
        n185 = call "CheckButtonPressed.vi"("Button"=w390) -> ("Pressed?"=w394:bool)  [unwired: 9 in, 1 out]
        n186 = case shown="True" w394 {
          tunnel: w398 -> [w416 _]
          tunnel: w397 -> [w415 _]
          tunnel: [w416 w417] -> w396
          tunnel: [w415 w417] -> w395
          frame False {
          }
          frame True {
            w417 = 0
          }
        }
        n187 = Or(x="Calibrate?", y=w390) -> (x .or. y?=w391:bool)
        n188 = case shown="True" w391 {
          tunnel: w407 -> [w428 w438]
          tunnel: [w428 w435] -> w406
          tunnel: w396 -> [w430 w444]
          tunnel: w395 -> [w431 w446]
          tunnel: w405 -> [w429 w447]
          tunnel: [w429 w434] -> w400
          tunnel: [w431 w445] -> w403
          tunnel: [w430 w443] -> w402
          tunnel: "Color Components" -> [_ w440]
          tunnel: "Color System" -> [_ w439]
          tunnel: "Calibrate?" -> [_ w437]
          tunnel: [_ w433] -> _
          tunnel: w388 -> [_ w432]
          frame False {
          }
          frame True {
            # "Process image"
            # "Increment number of hot\ngoals if hot"
            n189 = case shown="True" w437 {
              tunnel: w439 -> [_ w464]
              tunnel: w440 -> [_ w463]
              tunnel: w438 -> [_ w462]
              frame False {
              }
              frame True {
                w465 = cluster{"Hue":dbl, "Sat":dbl, "Val":dbl} {"Hue"=4.0, "Sat"=6.0, "Val"=4.0}  # Std Devs
                n190 = control-ref of="Camera Image"() -> (w461:refnum<vi>)
                n191 = call "Calibration Helper.vi"("Std Devs"=w465, "Color Mode"=w464, "Color Components"=w463, "Image"=w462, "Image Ctl Refnum"=w461) -> ("Changed"=w459:bool, "output color"=w460:T31)  [unwired: 5 in]
                n192 = case shown="True" w459 {
                  tunnel: w460 -> [_ w466]
                  frame False {
                  }
                  frame True {
                    n193 = local write "Color Components"(w466) -> ()
                  }
                }
              }
            }
            n194 = call-poly "CheckImagePoly.vi"("Score cutoff"="Score cutoff", "error in"=w447, "Color Components"=w440, "Color System"=w439, "Image"=w438) -> ("error out"=w434:errorcluster, "Hot?"=w441:bool, "Distance (ft)"=→"Distance (ft)":dbl, "Image out"=w435:T17)  [unwired: 3 in]
            n195 = Increment(x=w446) -> (x+1=w445:i32)
            n196 = case shown="True" w441 {
              tunnel: w444 -> [w467 w469]
              tunnel: [w467 w468] -> w443
              frame False {
              }
              frame True {
                n197 = Increment(x=w469) -> (x+1=w468:i32)
              }
            }
            n198 = case shown="True" "SaveCameraImage?" {
              tunnel: w435 -> [_ w458]
              tunnel: w434 -> [_ w457]
              tunnel: [_ w456] -> w433
              tunnel: w432 -> [_ w453]
              frame False {
              }
              frame True {
                n199 = call <vilib>:"Application Directory.vi"() -> ("Application Directory"=w449:path)
                n200 = Number To Decimal String(number=w453) -> (decimal integer string=w452:string)  [unwired: 1 in]
                n201 = Concatenate Strings("CameraImage", w452, ".jpg" ("string")) -> (w450:string)
                n202 = Build Path(base path=w449, name or relative path=w450) -> (appended path=w455:path)
                n203 = call-poly "IMAQ Write File 2"("error in (no error)"=w457, "File Path"=w455, "Image"=w458) -> ("error out"=w456:errorcluster)  [unwired: 7 in, 1 out]
              }
            }
          }
        }
        "Camera Image" <- w406
        "NumHot" <- w402
        "NumProcessed" <- w403
        n204 = Greater Or Equal?(x=w403, y="NumSamples") -> (x >= y?=w404:bool)
        n205 = case shown="True" w404 {
          tunnel: w402 -> [_ w425]
          tunnel: "NumSamples" -> [_ w426]
          frame False {
          }
          frame True {
            w418 = TRUE ("Finished?")
            # "Finished? must update\nbefore Hot?"
            # "Check if proportion\nis greater than cutoff %"
            n206 = local write "ProcessImage?"(FALSE ("ProcessImage?")) -> ()
            n207 = To Double Precision Float(number=w425) -> (double precision float=w423:dbl)
            n208 = To Double Precision Float(number=w426) -> (double precision float=w424:dbl)
            n209 = Divide(x=w423, y=w424) -> (x/y=w422:dbl)
            n210 = Greater Or Equal?(x=w422, y="% Cutoff") -> (x >= y?=w420:bool)
            n211 = case shown="True" w418 {
              tunnel: w420 -> [_ w427]
              frame False {
              }
              frame True {
                n212 = local write "Hot?"(w427) -> ()
              }
            }
            n213 = local write "Finished?"(w418) -> ()
          }
        }
        "Mbps" <- w409
        "fps" <- w408
      }
    }
    n214 = call "GetTime.vi"("error in"=w365) -> ("Time"=w367:u32)
    n215 = call "GetTime.vi"("error in"=w368) -> ("Time"=w369:u32)
    n216 = case shown="True" "Reset?" {
      tunnel: w363 -> [w381 _]
      tunnel: w362 -> [w382 _]
      tunnel: [w382 w383] -> w361
      tunnel: [w381 w383] -> w360
      frame False {
      }
      frame True {
        w383 = 0
      }
    }
    n217 = Subtract(x=w369, y=w367) -> (x-y=→"LoopTime":u32)
  }
  n218 = while {
    tunnel: w33 -> [w480]
    shift-right: [w479] -> _
    shift-left: w31 -> [w478]
    tunnel: [w477] -> _
    tunnel: w30 -> [w476]
    tunnel: w26 -> [w475]
    tunnel: w25 -> [w474]
    tunnel: w24 -> [_]
    tunnel: w18 -> [w473]
    i -> [w477]
    stop <- FALSE stop-if-true
    n219 = event shown="[0] Timeout" {
      selector: w474 -> [_ _ _ _ _ _ _ _ _ _ _ _ _ _ _ _]
      dyn-events: [_ _ _ _ _ _ _ _ _ _ _ _ _ w718 _ _] -> _
      timeout: u32 60 ("milliseconds to wait") -> [_ _ _ _ _ _ _ _ _ _ _ _ _ _ _ _]
      tunnel: w476 -> [w490 _ _ _ _ _ _ _ _ _ _ _ _ _ _ _]
      tunnel: "Test Tree" -> [_ _ _ _ _ _ _ _ w687 w695 w697 w701 w709 _ _ _]
      tunnel: w480 -> [_ w514 _ _ _ _ w651 w681 _ _ _ _ _ _ _ _]
      tunnel: [w484 w513 w612 w617 w625 w637 w650 w674 w686 w693 w696 w700 w708 w720 w734 w735] -> w479
      tunnel: w478 -> [w484 w513 w612 w617 w625 w637 w649 w674 w686 w693 w696 w700 w708 w720 w734 w735]
      tunnel: w475 -> [_ _ _ _ _ _ _ _ _ _ _ _ _ w721 _ w738]
      tunnel: w473 -> [_ _ _ _ _ _ _ _ _ _ _ _ _ w716 _ _]
      event Timeout {
        w489 = enum16{"Update", "Clear"}[] [enum."Clear", enum."Clear", enum."Clear", enum."Clear", enum."Update", enum."Update", enum."Clear"] items=["Update", "Clear"]
        n220 = event-data() -> ()  [unwired: 1 in, 1 out]
        n221 = local read "Mode"() -> (w487:T8)
        n222 = Index Array(array=w489, index=w487) -> (element=w488:enum16{"Update", "Clear"})
        n223 = call <vilib>:"NT Read String.vi"("Name"="TestMode/TestName") -> ("String"=w493:string)  [unwired: 9 in, 1 out]
        n224 = case shown="\"Variables\"" "Dashboard Tab" {
          tunnel: w490 -> [_ w503 _]
          tunnel: "/TestMode/Automatic/" ("Name Pattern") -> [_ w502 _]
          tunnel: w488 -> [_ w501 _]
          tunnel: w487 -> [_ w499 _]
          tunnel: [_ _ w505] -> _
          frame "Auto", Default {
          }
          frame "Test" {
            w498 = -2 ("Active Item:Row Number")
            n225 = call <vilib>:"NT Read and Format Entries as Tree.vi"("Operation"=w501, "Name Pattern"=w502, "Tree Refnum"=w503) -> ()  [unwired: 7 in, 2 out]
            n226 = Index Array(array=u32[] [14013909, 14013909, 14013909, 14013909, 14013909, 16777215, 14013909], index=w499) -> (element=w497:u32)
            n227 = property on="Test Tree" class="Tree (strict)"("Active Item Row Number"=w498, "ActiveColNum"=w498, "CellBG"=w497, "Active Item Row Number"=-1 ("Active Item:Row Number"), "CellBG"=u32 5789784 ("Color Box")) -> ()  [unwired: 2 in, 2 out]
          }
          frame "Variables" {
            n228 = control-ref of="Tree"() -> (w504:refnum<vi>)
            n229 = call <vilib>:"NT Read and Format Entries as Tree.vi"("Tree Refnum"=w504) -> ("Formatted Strings"=w505:cluster{"Name":string, "Value":string}[])  [unwired: 9 in, 1 out]
          }
        }
        n230 = case shown="Default" w493 {
          tunnel: "TestMode/TestProgress" ("Name") -> [w507 _]
          tunnel: "TestMode/TestProgressText" ("Name") -> [w506 _]
          frame Default {
            n231 = call <vilib>:"NT Read Number.vi"("Name"=w507) -> ("Numeric"=w508:dbl)  [unwired: 9 in, 1 out]
            n232 = call <vilib>:"NT Read String.vi"("Name"=w506) -> ("String"=w509:string)  [unwired: 9 in, 1 out]
            n233 = Bundle("Numeric"=w508, "String"=w509) -> (→"Progress":cluster{"Numeric":dbl, "String":string})  [unwired: 1 in]
          }
          frame "" {
            n234 = property on="Progress" class="Clust (strict)"("Visible"=FALSE) -> ()  [unwired: 2 in, 2 out]
            n235 = local write "Test Name"(u16 0) -> ()
          }
        }
      }
      event "Test Tree": Value Change {
        # "Show appropriate\ncontrols"
        n236 = event-data() -> ("CtlRef"=w517:refnum<vi>, "NewVal"=w515:string)  [unwired: 1 in]
        n237 = call <vilib>:"WPI_UtilitiesGetTreeIOName.vi"("NewVal"=w515, "TreeControl in"=w517) -> ("I/O Name"=w518:string)  [unwired: 9 in]
        n238 = case shown="\"Camera\"" w518 {
          selector: w518 -> [_ w525 _ w543 w552 _]
          tunnel: w515 -> [_ _ w540 w542 _ w559]
          tunnel: w514 -> [_ _ _ _ _ w558]
          frame Default {
            w520 = FALSE ("Visible")
            w519 = FALSE ("Visible")
            n239 = property on="Motor" class="Clust (strict)"("Visible"=w519) -> ()  [unwired: 2 in, 2 out]
            n240 = property on="Test Ring" class="Ring (strict)"("Visible"=w519) -> ()  [unwired: 2 in, 2 out]
            n241 = property on="Rev/Fwd" class="Clust (strict)"("Visible"=w520) -> ()  [unwired: 2 in, 2 out]
            n242 = property on="On/Off" class="Bool (strict)"("Visible"=w520) -> ()  [unwired: 2 in, 2 out]
            n243 = property on="Test Slider" class="Slide (strict)"("Visible"=w520) -> ()  [unwired: 2 in, 2 out]
          }
          frame "Motor", "PWM" {
            w526 = FALSE ("Visible")
            n244 = case shown="\"Motor\", Default" w525 {
              tunnel: [1.0 ("Value") -1.0 ("Value")] -> w524
              tunnel: [255.0 ("Value") 1.0 ("Value")] -> w523
              tunnel: [128.0 ("Value") 0.0 ("Value")] -> w522
              tunnel: [64.0 ("Value") 0.5 ("Value")] -> w521
              frame "PWM" {
              }
              frame "Motor", Default {
              }
            }
            n245 = property on="Motor" class="Clust (strict)"("Visible"=TRUE) -> ()  [unwired: 2 in, 2 out]
            n246 = property on="Value" class="Slide (strict)"("Value"=w522, "Scale.Minimum"=w524, "Scale.Maximum"=w523, "Scale.Increment"=w521) -> ()  [unwired: 2 in, 2 out]
            n247 = property on="On/Off" class="Bool (strict)"("Visible"=w526) -> ()  [unwired: 2 in, 2 out]
            n248 = property on="Test Slider" class="Slide (strict)"("Visible"=w526) -> ()  [unwired: 2 in, 2 out]
            n249 = property on="Test Ring" class="Ring (strict)"("Visible"=w526) -> ()  [unwired: 2 in, 2 out]
            n250 = property on="Rev/Fwd" class="Clust (strict)"("Visible"=w526) -> ()  [unwired: 2 in, 2 out]
          }
          frame "Servo" {
            w538 = FALSE ("Visible")
            n251 = call <vilib>:"NT Read Number.vi"("Name"=w540) -> ("Numeric"=w539:dbl)  [unwired: 9 in, 1 out]
            n252 = property on="Test Slider" class="Slide (strict)"("Visible"=TRUE, "Scale.Maximum"=170.0 ("Scale.Range:Maximum")) -> ()  [unwired: 2 in, 2 out]
            n253 = local write "Test Slider"(w539) -> ()
            n254 = property on="Motor" class="Clust (strict)"("Visible"=w538) -> ()  [unwired: 2 in, 2 out]
            n255 = property on="Rev/Fwd" class="Clust (strict)"("Visible"=w538) -> ()  [unwired: 2 in, 2 out]
            n256 = property on="On/Off" class="Bool (strict)"("Visible"=w538) -> ()  [unwired: 2 in, 2 out]
            n257 = property on="Test Ring" class="Ring (strict)"("Visible"=w538) -> ()  [unwired: 2 in, 2 out]
          }
          frame "Relay", "Solenoid" {
            w541 = FALSE ("Visible")
            n258 = property on="Motor" class="Clust (strict)"("Visible"=w541) -> ()  [unwired: 2 in, 2 out]
            n259 = property on="Test Slider" class="Slide (strict)"("Visible"=w541) -> ()  [unwired: 2 in, 2 out]
            n260 = Search and Replace String(input string=w542, search string="/Value  **", replace string="/Direction") -> (result string=w548:string)  [unwired: 5 in, 3 out]
            n261 = property on="Test Ring" class="Ring (strict)"("Visible"=w541) -> ()  [unwired: 2 in, 2 out]
            n262 = call <vilib>:"NT Read String.vi"("Name"=w548) -> ("String"=w546:string)  [unwired: 9 in, 1 out]
            n263 = Equal?(x="Both directions", y=w546) -> (x = y?=w544:bool)
            n264 = Not(x=w544) -> (.not. x?=w545:bool)
            n265 = property on="Rev/Fwd" class="Clust (strict)"("Visible"=w544) -> ()  [unwired: 2 in, 2 out]
            n266 = property on="On/Off" class="Bool (strict)"("Visible"=w545, "Caption.Text"=w543) -> ()  [unwired: 2 in, 2 out]
          }
          frame "Compressor", "Digital Out" {
            w551 = FALSE ("Visible")
            # "Get direction and finish"
            n267 = property on="Motor" class="Clust (strict)"("Visible"=w551) -> ()  [unwired: 2 in, 2 out]
            n268 = property on="Test Slider" class="Slide (strict)"("Visible"=w551) -> ()  [unwired: 2 in, 2 out]
            n269 = property on="Test Ring" class="Ring (strict)"("Visible"=w551) -> ()  [unwired: 2 in, 2 out]
            n270 = property on="On/Off" class="Bool (strict)"("Visible"=TRUE, "Caption.Text"=w552) -> ()  [unwired: 2 in, 2 out]
            n271 = property on="Rev/Fwd" class="Clust (strict)"("Visible"=FALSE) -> ()  [unwired: 2 in, 2 out]
          }
          frame "Camera" {
            n272 = call <vilib>:"Get Last Path Segment.vi"("String in"=w559) -> ("String out"=w560:string)  [unwired: 10 in]
            n273 = property on="On/Off" class="Bool (strict)"("Visible"=FALSE) -> ()  [unwired: 2 in, 2 out]
            n274 = property on="Motor" class="Clust (strict)"("Visible"=FALSE) -> ()  [unwired: 2 in, 2 out]
            n275 = property on="Rev/Fwd" class="Clust (strict)"("Visible"=FALSE) -> ()  [unwired: 2 in, 2 out]
            n276 = case shown="\"White Balance  **\"" w560 {
              tunnel: w559 -> [w566 w575 w584 w593 w602 _ w608]
              tunnel: w558 -> [w564 w572 w581 w590 w599 _ _]
              frame "Size  **" {
                n277 = Index Array(array=w564) -> (element=w563:cluster{string[]})  [unwired: 1 in]
                n278 = call <vilib>:"NT Read String.vi"("Name"=w566) -> ("String"=w565:string)  [unwired: 9 in, 1 out]
                n279 = Unbundle(w563) -> (w561:string[])
                n280 = Match First String(2:w561, 3:w565) -> (0:w562:i32)  [unwired: 1 out]
                n281 = property on="Test Ring" class="Ring (strict)"("Value"=w562, "Strings []"=w561) -> ()  [unwired: 2 in, 2 out]
                n282 = property on="Test Ring" class="Ring (strict)"("Visible"=TRUE) -> ()  [unwired: 2 in, 2 out]
                n283 = property on="Test Slider" class="Slide (strict)"("Visible"=FALSE) -> ()  [unwired: 2 in, 2 out]
              }
              frame "White Balance  **" {
                n284 = Index Array(array=w572, index=1) -> (element=w573:cluster{string[]})
                n285 = call <vilib>:"NT Read String.vi"("Name"=w575) -> ("String"=w574:string)  [unwired: 9 in, 1 out]
                n286 = Unbundle(w573) -> (w570:string[])
                n287 = Match First String(2:w570, 3:w574) -> (0:w569:i32)  [unwired: 1 out]
                n288 = property on="Test Ring" class="Ring (strict)"("Value"=w569, "Strings []"=w570) -> ()  [unwired: 2 in, 2 out]
                n289 = property on="Test Ring" class="Ring (strict)"("Visible"=TRUE) -> ()  [unwired: 2 in, 2 out]
                n290 = property on="Test Slider" class="Slide (strict)"("Visible"=FALSE) -> ()  [unwired: 2 in, 2 out]
              }
              frame "Exposure  **" {
                n291 = Index Array(array=w581, index=2) -> (element=w582:cluster{string[]})
                n292 = call <vilib>:"NT Read String.vi"("Name"=w584) -> ("String"=w583:string)  [unwired: 9 in, 1 out]
                n293 = Unbundle(w582) -> (w578:string[])
                n294 = Match First String(2:w578, 3:w583) -> (0:w579:i32)  [unwired: 1 out]
                n295 = property on="Test Ring" class="Ring (strict)"("Value"=w579, "Strings []"=w578) -> ()  [unwired: 2 in, 2 out]
                n296 = property on="Test Ring" class="Ring (strict)"("Visible"=TRUE) -> ()  [unwired: 2 in, 2 out]
                n297 = property on="Test Slider" class="Slide (strict)"("Visible"=FALSE) -> ()  [unwired: 2 in, 2 out]
              }
              frame "Exposure Priority  **" {
                n298 = Index Array(array=w590, index=3) -> (element=w591:cluster{string[]})
                n299 = call <vilib>:"NT Read String.vi"("Name"=w593) -> ("String"=w592:string)  [unwired: 9 in, 1 out]
                n300 = Unbundle(w591) -> (w587:string[])
                n301 = Match First String(2:w587, 3:w592) -> (0:w588:i32)  [unwired: 1 out]
                n302 = property on="Test Ring" class="Ring (strict)"("Value"=w588, "Strings []"=w587) -> ()  [unwired: 2 in, 2 out]
                n303 = property on="Test Ring" class="Ring (strict)"("Visible"=TRUE) -> ()  [unwired: 2 in, 2 out]
                n304 = property on="Test Slider" class="Slide (strict)"("Visible"=FALSE) -> ()  [unwired: 2 in, 2 out]
              }
              frame "Color Enable  **" {
                n305 = Index Array(array=w599, index=4) -> (element=w600:cluster{string[]})
                n306 = call <vilib>:"NT Read String.vi"("Name"=w602) -> ("String"=w601:string)  [unwired: 9 in, 1 out]
                n307 = Unbundle(w600) -> (w596:string[])
                n308 = Match First String(2:w596, 3:w601) -> (0:w597:i32)  [unwired: 1 out]
                n309 = property on="Test Ring" class="Ring (strict)"("Value"=w597, "Strings []"=w596) -> ()  [unwired: 2 in, 2 out]
                n310 = property on="Test Ring" class="Ring (strict)"("Visible"=TRUE) -> ()  [unwired: 2 in, 2 out]
                n311 = property on="Test Slider" class="Slide (strict)"("Visible"=FALSE) -> ()  [unwired: 2 in, 2 out]
              }
              frame Default {
                n312 = property on="Test Ring" class="Ring (strict)"("Visible"=FALSE) -> ()  [unwired: 2 in, 2 out]
                n313 = property on="Test Slider" class="Slide (strict)"("Visible"=FALSE) -> ()  [unwired: 2 in, 2 out]
              }
              frame "Brightness  **", "Color Level  **", "Compression  **", "FPS  **", "Sharpness  **" {
                n314 = call <vilib>:"NT Read Number.vi"("Name"=w608) -> ("Numeric"=w607:dbl)  [unwired: 9 in, 1 out]
                n315 = local write "Test Slider"(w607) -> ()
                n316 = property on="Test Slider" class="Slide (strict)"("Visible"=TRUE, "Scale.Maximum"=100.0 ("Scale.Range:Maximum")) -> ()  [unwired: 2 in, 2 out]
                n317 = property on="Test Ring" class="Ring (strict)"("Visible"=FALSE) -> ()  [unwired: 2 in, 2 out]
              }
            }
          }
        }
        n318 = property on="Progress" class="Clust (strict)"("Visible"=FALSE) -> ()  [unwired: 2 in, 2 out]
      }
      event "Test Name": Mouse Enter {
        # "Populate the ring with the list of tests"
        n319 = event-data() -> ()  [unwired: 1 in, 1 out]
        n320 = call <vilib>:"NT Read String Array.vi"("Name"="TestMode/TestList") -> ("String Array"=w616:string[])  [unwired: 9 in, 1 out]
        n321 = Build Array (concatenate)("Select the test to run...", w616) -> (w615:string[])
        n322 = property on="Test Name" class="Ring (strict)"("Strings []"=w615) -> ()  [unwired: 2 in, 2 out]
      }
      event "Test Name": Value Change {
        w618 = FALSE ("Visible")
        # "Tell the robot the test name to run"
        n323 = event-data() -> ("NewVal"=w622:u16)  [unwired: 1 in]
        n324 = property on="Test Name" class="Ring (strict)"() -> ("Strings []"=w623:string[])  [unwired: 2 in, 2 out]
        n325 = local write "Progress"(T18 {"Test Progress"=0, "Test Progress Text"=""} ("Progress")) -> ()
        n326 = Index Array(array=w623, index=w622) -> (element=w621:string)
        n327 = call <vilib>:"NT Write String.vi"("String"=w621, "Name"="TestMode/TestName") -> ()  [unwired: 9 in, 1 out]
        n328 = property on="Progress" class="Clust (strict)"("Visible"=TRUE) -> ()  [unwired: 2 in, 2 out]
        n329 = property on="Motor" class="Clust (strict)"("Visible"=w618) -> ()  [unwired: 2 in, 2 out]
        n330 = property on="Test Slider" class="Slide (strict)"("Visible"=w618) -> ()  [unwired: 2 in, 2 out]
        n331 = property on="On/Off" class="Bool (strict)"("Visible"=w618) -> ()  [unwired: 2 in, 2 out]
        n332 = property on="Rev/Fwd" class="Clust (strict)"("Visible"=w618) -> ()  [unwired: 2 in, 2 out]
        n333 = property on="Test Ring" class="Ring (strict)"("Visible"=w618) -> ()  [unwired: 2 in, 2 out]
      }
      event "Listbox": Double Click {
        n334 = event-data() -> ("PlatMods.Shift"=w626:bool, "Row"=w628:i32)  [unwired: 1 in]
        n335 = case shown="True" w626 {
          tunnel: w628 -> [w632 _]
          tunnel: 1 -> [w631 _]
          frame False {
            n336 = property on="Listbox" class="LstBox (strict)"() -> ("Item Symbols"=w630:i32[])  [unwired: 2 in, 2 out]
            n337 = Replace Array Subset(array=w630, new element=w631, index=w632) -> (w629:i32[])
            n338 = property on="Listbox" class="LstBox (strict)"("Item Symbols"=w629) -> ()  [unwired: 2 in, 2 out]
          }
          frame True {
            w633 = 0 ("Top Row")
            n339 = property on="Listbox" class="LstBox (strict)"() -> ("Number of Rows"=w635:u32)  [unwired: 2 in, 2 out]
            n340 = Initialize Array(0, w635) -> (w634:i32[])
            n341 = property on="Listbox" class="LstBox (strict)"("Top Row"=w633, "Value"=w633, "Item Symbols"=w634) -> ()  [unwired: 2 in, 2 out]
          }
        }
      }
      event "Listbox": Key Down {
        n342 = event-data() -> ("VKey"=w639:T32)  [unwired: 1 in]
        n343 = case shown="\"Left\", \"Right\"" w639 {
          selector: w639 -> [w644 _]
          tunnel: eventvkey."Left" ("VKey") -> [w642 _]
          frame "Left", "Right" {
            n344 = Equal?(x=w642, y=w644) -> (x = y?=w643:bool)
            n345 = Select(t=0, s=w643, f=1) -> (s? t:f=w645:i32)
            n346 = property on="Listbox" class="LstBox (strict)"() -> ("Item Symbols"=w648:i32[])  [unwired: 2 in, 2 out]
            n347 = Replace Array Subset(array=w648, new element=w645, index="Listbox") -> (w647:i32[])
            n348 = property on="Listbox" class="LstBox (strict)"("Item Symbols"=w647) -> ()  [unwired: 2 in, 2 out]
          }
          frame Default {
          }
        }
      }
      event "DB Camera Config": Value Change {
        n349 = event-data() -> ("NewVal"=w652:bool)  [unwired: 1 in]
        n350 = case shown="False" w652 {
          tunnel: w651 -> [w661 _]
          tunnel: [w654 w672] -> w650
          tunnel: w649 -> [w653 w672]
          frame False {
            w668 = "Camera"
            w671 = FALSE ("Visible")
            n351 = local read "Camera Settings"() -> (w660:T7)
            n352 = Index Array(array=w661) -> (element=w664:cluster{string[]})  [unwired: 1 in]
            n353 = Unbundle(w660) -> ("Frame Rate"=w659:i32, "Compression"=w658:i32, "Size"=w662:u16)
            n354 = Unbundle(w664) -> (w663:string[])
            n355 = Index Array(array=w663, index=w662) -> (element=w657:string)
            n356 = call-poly <vilib>:"Write Key.vi"("section"=w668, "value"=w657, "key"="Size", "refnum"=w653) -> ("refnum out"=w670:T25)  [unwired: 2 in, 5 out]
            n357 = call-poly <vilib>:"Write Key.vi"("section"=w668, "value"=w659, "key"="FrameRate", "refnum"=w670) -> ("refnum out"=w669:T25)  [unwired: 1 in, 6 out]
            n358 = property on="Camera Settings" class="Clust (strict)"("Visible"=w671) -> ()  [unwired: 2 in, 2 out]
            n359 = local write "DB Camera Config"(w671) -> ()
            n360 = call-poly <vilib>:"Write Key.vi"("section"=w668, "value"=w658, "key"="Compression", "refnum"=w669) -> ("refnum out"=w655:T25)  [unwired: 1 in, 6 out]
            n361 = call <vilib>:"Close Config Data.vi"("refnum"=w655) -> ("file path"=w656:path)  [unwired: 2 in, 8 out]
            n362 = call <vilib>:"Open Config Data.vi"("configuration file path"=w656) -> ("refnum"=w654:T25)  [unwired: 8 in, 2 out]
          }
          frame True {
            n363 = property on="Camera Settings" class="Clust (strict)"("Visible"=TRUE) -> ()  [unwired: 2 in, 2 out]
          }
        }
      }
      event "Camera Settings": Value Change {
        n364 = event-data() -> ("NewVal"=w685:T7)  [unwired: 1 in]
        n365 = Index Array(array=w681) -> (element=w680:cluster{string[]})  [unwired: 1 in]
        n366 = Unbundle(w685) -> ("Frame Rate"=w676:i32, "Compression"=w675:i32, "Size"=w678:u16)
        n367 = Unbundle(w680) -> (w679:string[])
        n368 = Index Array(array=w679, index=w678) -> (element=w677:string)
        n369 = Format Into String(format string="%s   %dfps   %d%%", w677, w676, w675) -> (resulting string=w682:string)  [unwired: 2 in, 1 out]
        n370 = Build Array(w682) -> (w683:string[])
        n371 = property on="DB Camera Config" class="Bool (strict)"("Strings [4]"=w683) -> ()  [unwired: 2 in, 2 out]
      }
      event "Motor.Enable": Value Change {
        n372 = event-data() -> ("NewVal"=w691:bool)  [unwired: 1 in]
        n373 = Unbundle("Motor") -> ("Value"=w690:dbl)  [unwired: 1 out]
        n374 = Select(t=w690, s=w691, f=0.0) -> (s? t:f=w688:dbl)
        n375 = call <vilib>:"NT Write Number.vi"("Numeric"=w688, "Name"=w687) -> ()  [unwired: 9 in, 1 out]
      }
      event "Test Slider": Value Change {
        n376 = event-data() -> ("NewVal"=w694:dbl)  [unwired: 1 in]
        n377 = call <vilib>:"NT Write Number.vi"("Numeric"=w694, "Name"=w695) -> ()  [unwired: 9 in, 1 out]
      }
      event "On/Off": Value Change {
        n378 = event-data() -> ("NewVal"=w699:bool)  [unwired: 1 in]
        n379 = Boolean To (0,1)(Boolean=w699) -> (0, 1=w698:i16)
        n380 = call <vilib>:"NT Write Number.vi"("Numeric"=w698, "Name"=w697) -> ()  [unwired: 9 in, 1 out]
      }
      event "Rev/Fwd": Value Change {
        n381 = event-data() -> ("NewVal.Forward"=w707:bool, "NewVal.Reverse"=w706:bool)  [unwired: 1 in]
        n382 = Boolean To (0,1)(Boolean=w707) -> (0, 1=w703:i16)
        n383 = Boolean To (0,1)(Boolean=w706) -> (0, 1=w705:i16)
        n384 = Negate(x=w705) -> (-x=w704:i16)
        n385 = Add(x=w703, y=w704) -> (x+y=w702:i16)
        n386 = call <vilib>:"NT Write Number.vi"("Numeric"=w702, "Name"=w701) -> ()  [unwired: 9 in, 1 out]
      }
      event "Test Ring": Value Change {
        n387 = event-data() -> ("NewVal"=w711:u16)  [unwired: 1 in]
        n388 = property on="Test Ring" class="Ring (strict)"() -> ("Strings []"=w712:string[])  [unwired: 2 in, 2 out]
        n389 = Index Array(array=w712, index=w711) -> (element=w710:string)
        n390 = call <vilib>:"NT Write String.vi"("String"=w710, "Name"=w709) -> ()  [unwired: 9 in, 1 out]
      }
      event "Rec Mode": Value Change {
        # "Update globals for recording mode and path to read log from.\nClear when logging and let NetworkTables set path for vision to\nuse."
        n391 = event-data() -> ("NewVal"=w722:enum32{"Stop", "Record", "Playback"})  [unwired: 1 in]
        n392 = global write "WPI_DashboardLogging Global.vi" "Logging Filename"(path "") -> ()
        n393 = case shown="\"Stop\", \"Record\"" w722 {
          tunnel: w721 -> [_ w724 w732]
          tunnel: [_ _ w731] -> w718
          tunnel: [_ _ w730] -> _
          tunnel: w716 -> [_ _ w728]
          tunnel: cluster{i32, i32} {-250, 170} -> [_ _ w727]
          tunnel: [_ _ T33 {"Image Size"=TRUE, "Image Type"=TRUE, "Pixel Value"=TRUE, "ROI Information"=TRUE, "Zoom Factor"=FALSE} ("Image Information Shown:All Elements")] -> w714
          tunnel: [_ _ TRUE ("Zoom Factor")] -> w713
          frame Default {
          }
          frame "Stop", "Record" {
            # "Place Window too"
            n394 = invoke class="VI" method="FP.Close"(reference=w724) -> (reference out=w723:refnum<vi>)  [unwired: 2 in, 2 out]
            n395 = invoke class="VI" method="Abort VI"(reference=w723) -> ()  [unwired: 2 in, 3 out]
          }
          frame "Playback" {
            n396 = call "Open Playback Panel.vi"("Offset"=w727, "DB VI Ref"=w728, "Playback in"=w732) -> ("Playback out"=w729:refnum<vi>)  [unwired: 8 in]
            n397 = register-events(w729) -> (reference out=w731:refnum<event-registration>, error out=w730:errorcluster)  [unwired: 2 in]
          }
        }
        n398 = global write "WPI_DashboardLogging Global.vi" "Recording"(w722) -> ()
        n399 = property on="Camera Image" class="ImageControl"("Image Information Shown"=w714, "Image Information Visible"=w713) -> ()  [unwired: 2 in, 2 out]
        n400 = call <vilib>:"WPI_DashboardNT Log FieldName Cache.vi"("Operation"=enum16{"Lookup/Add", "Index", "Clear"}."Clear") -> ()  [unwired: 8 in, 3 out]
      }
      event Panel Close {
        w733 = enum32{"Stop", "Record", "Playback"}."Stop" ("Rec Mode")
        n401 = event-data() -> ()  [unwired: 1 in, 4 out]
        n402 = local write "Rec Mode"(w733) -> ()
        n403 = global write "WPI_DashboardLogging Global.vi" "Recording"(w733) -> ()
      }
      event Panel Close {
        # "Abort playback window and ourself"
        n404 = event-data() -> ()  [unwired: 1 in, 4 out]
        n405 = invoke class="VI" method="FP.Close"(reference=w738) -> (reference out=w737:refnum<vi>)  [unwired: 2 in, 2 out]
        n406 = invoke class="VI" method="Abort VI"(reference=w737) -> (error out=w736:errorcluster)  [unwired: 2 in, 2 out]
        n407 = invoke class="VI" method="Abort VI"(error in=w736) -> ()  [unwired: 2 in, 3 out]
      }
    }
  }
  n408 = property on="On/Off" class="Bool (strict)"("Visible"=w34) -> ()  [unwired: 2 in, 2 out]
  n409 = property on="Motor" class="Clust (strict)"("Visible"=w34) -> ()  [unwired: 2 in, 2 out]
  n410 = property on="Progress" class="Clust (strict)"("Visible"=w34) -> ()  [unwired: 2 in, 2 out]
  n411 = property on="Test Ring" class="Ring (strict)"("Visible"=w34) -> ()  [unwired: 2 in, 2 out]
  n412 = property on="Rev/Fwd" class="Clust (strict)"("Visible"=w34) -> ()  [unwired: 2 in, 2 out]
  n413 = property on="Camera Settings" class="Clust (strict)"("Visible"=w34) -> ()  [unwired: 2 in, 2 out]
  n414 = local write "DB Camera Config"(w34) -> ()
  n415 = global write "WPI_DashboardLogging Global.vi" "Recording"(w19) -> ()
  n416 = local write "Rec Mode"(w19) -> ()
